vi "Unpack for gRPC.vi"(8 "error in":errorcluster, 9 "configuration / results":enum16{"Configuration", "Results"}(ring), 10 "any":T1, 11 "measurement customizations in":refnum<class "Measurement Plugin.lvclass">) -> (0 "error out":errorcluster, 2 "data value":variant, 3 "measurement customizations out":refnum<class "Measurement Plugin.lvclass">)   [LabVIEW 2024, in "Device Power Sequencer.lvlib" / "Measurement Plugin.lvclass"]
uses:
  Measurement Plugin.lvclass
  Measurement Plugin.lvclass/Measurement Plugin.ctl
  Measurement Configuration.ctl
  Device Power Sequencer.lvlib
  Measurement Results.ctl
  3ecd018e-d556-4cbc-bc60-c4ba57204520.vi
  a521b266-ce99-437c-923d-067dcf1e07fd.vi
  <vilib>/Plug-In SDKs/Measurements/Measurement Plugin Service/Measurement Plugin Service.lvclass
  controls/Power line frequency.ctl
  controls/Transient Response.ctl
  controls/Relative To.ctl
  controls/Sense Mode.ctl
  controls/Source Mode.ctl
  C:/Program Files/National Instruments/LabVIEW 2024/vi.lib/Plug-In SDKs/Measurements/Measurement Plugin Service/Measurement Plugin Service.lvclass
  C:/dev/device-power-sequencer/source/Device Power Sequencer/Advanced/Measurement Plugin.lvclass
  <vilib>/gRPC/LabVIEW gRPC Library/Shared/Any.ctl
  <vilib>/gRPC/LabVIEW gRPC Library/grpc-lvsupport-release.lvlib
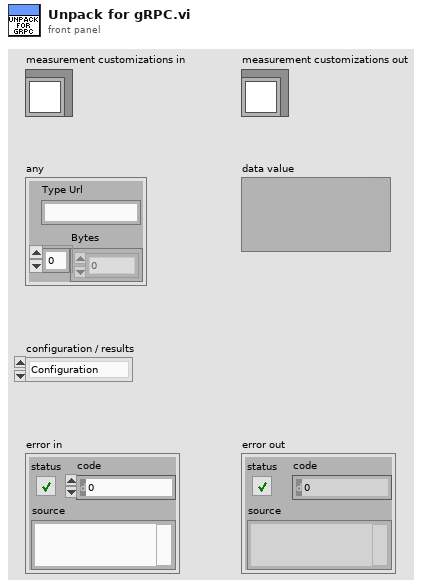
[diagram p1: front panel]
types:
  T1 = typedef "grpc-lvsupport-release.lvlib/Any.ctl" = cluster{"Type Url":string, "Bytes":u8[]}
  T2 = typedef "grpc-lvsupport-release.lvlib/grpcId.ctl" = u64
  T3 = typedef "Device Power Sequencer.lvlib/Measurement Configuration.ctl" = cluster{"Quick Power Down":bool, "Pin Name":string[], "Source Mode":T4[], "Start Value":dbl[], "Target Value":dbl[], "Compliance Limit":dbl[], "Sense Mode":T5[], "Default Ramp Rate":bool[], "Ramp Rate":dbl[], "Start Delay":dbl[], "Relative To":T6[], "Transient Response":T7[], "Data Capture":bool, "Power line frequency":T8}
  T4 = typedef "Device Power Sequencer.lvlib/Source Mode.ctl" = i32
  T5 = typedef "Device Power Sequencer.lvlib/Sense Mode.ctl" = i32
  T6 = typedef "Device Power Sequencer.lvlib/Relative To.ctl" = u32
  T7 = typedef "Device Power Sequencer.lvlib/Transient Response.ctl" = i32
  T8 = typedef "Device Power Sequencer.lvlib/Power line frequency.ctl" = u32
  T9 = typedef "Device Power Sequencer.lvlib/Measurement Results.ctl" = cluster{"Voltage Measurements":dbl[], "Current Measurements":dbl[], "Indices":i32[], "dt values":dbl[], "Default Ramp Rate?":bool[], "Actual Ramp Rates":dbl[], "Warning":string[], "Operation Complete?":bool}
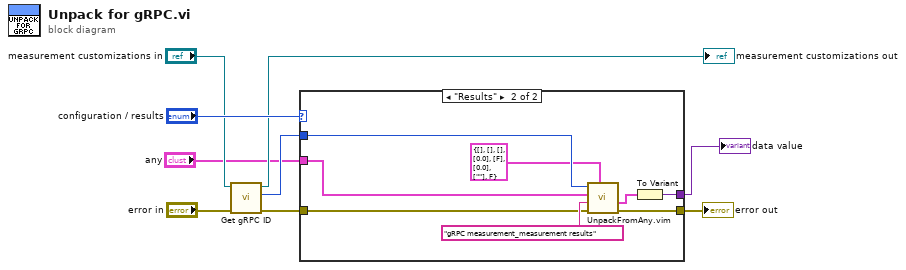
[diagram p0: block diagram]
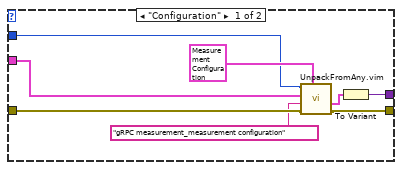
[diagram p2: hidden frame]
diagram:
  n1 = call <vilib>:"Get gRPC ID.vi"("error in"="error in", "measurement plugin service in"="measurement customizations in") -> ("error out"=w6:errorcluster, "gRPC ID"=w3:T2, "measurement plugin service out"=→"measurement customizations out":refnum<class "Measurement Plugin.lvclass">)  [unwired: 7 in]
  n2 = case shown="\"Results\"" "configuration / results" {
    tunnel: w6 -> [w15 w19]
    tunnel: "any" -> [w10 w18]
    tunnel: w3 -> [w12 w22]
    tunnel: [w16 w23] -> w9
    tunnel: [w17 w25] -> w1
    frame "Configuration" {
      n3 = call "UnpackFromAny.vim"("Data Type"=T3 {"Quick Power Down"=TRUE, "Pin Name"=[], "Source Mode"=[0, 0], "Start Value"=[0.0, 0.0], "Target Value"=[0.0, 0.0], "Compliance Limit"=[0.0, 0.0], "Sense Mode"=[], "Default Ramp Rate"=[], "Ramp Rate"=[], "Start Delay"=[], "Relative To"=[], "Transient Response"=[], "Data Capture"=FALSE, "Power line frequency"=32} ("Measurement Configuration"), "error in"=w15, "Message Type"="gRPC measurement_measurement configuration", "Any"=w10, "gRPCid in"=w12) -> ("error out"=w16:errorcluster, "Unpacked Value"=w14:T3)  [unwired: 4 in, 1 out]
      n4 = To Variant(anything=w14) -> (Variant=w17:variant)
    }
    frame "Results" {
      n5 = call "UnpackFromAny.vim"("Data Type"=T9 {"Voltage Measurements"=[], "Current Measurements"=[], "Indices"=[], "dt values"=[0.0], "Default Ramp Rate?"=[FALSE], "Actual Ramp Rates"=[0.0], "Warning"=[""], "Operation Complete?"=FALSE} ("Measurement Results"), "error in"=w19, "Message Type"="gRPC measurement_measurement results", "Any"=w18, "gRPCid in"=w22) -> ("error out"=w23:errorcluster, "Unpacked Value"=w24:T9)  [unwired: 4 in, 1 out]
      n6 = To Variant(anything=w24) -> (Variant=w25:variant)
    }
  }
  "error out" <- w9
  "data value" <- w1
